vi "Write Cache.vi"(8 "error in (no error)":errorcluster, 10 "Cache":variant, 11 "App Control API in":refnum<class "AppControlAPI.lvclass">) -> (0 "error out":errorcluster, 3 "App Control API out":refnum<class "AppControlAPI.lvclass">)   [LabVIEW 2018, in "AppControlAPI.lvclass"]
uses:
  AppControlAPI.lvclass
  AppControlAPI.lvclass/AppControlAPI.ctl
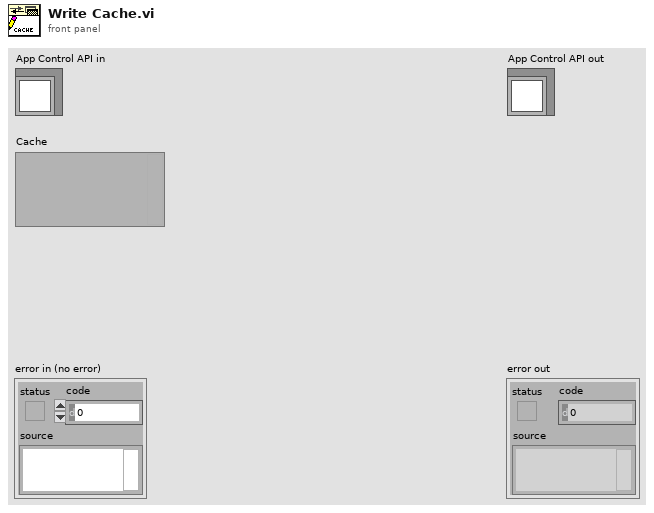
[diagram p1: front panel]
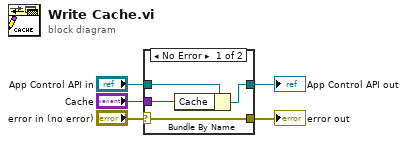
[diagram p0: block diagram]
diagram:
  n1 = case shown="No Error" "error in (no error)" {
    selector: "error in (no error)" -> [w9 w10]
    tunnel: [w9 w10] -> w4
    tunnel: [w7 w11] -> w2
    tunnel: "App Control API in" -> [w8 w11]
    tunnel: "Cache" -> [w6 _]
    frame No Error {
      n2 = Bundle By Name(cluster=w8, "Cache"=w6) -> (w7:refnum<class "AppControlAPI.lvclass">)
    }
    frame Error {
    }
  }
  "error out" <- w4
  "App Control API out" <- w2
